vi "First Check.vi"(8 "error in (no error)":errorcluster) -> (0 "error out":errorcluster)   [LabVIEW 2023, in "Heart.lvlib"]
uses:
  Heart.lvlib
  <vilib>/xnet/xnet.llb/XNET Frame CAN.ctl
  <vilib>/xnet/xnet.llb/XNET Frame Type CAN.ctl
  <vilib>/xnet/xnet.llb/XNET Create Session (Frame Output Single-point).vi
  <vilib>/xnet/xnet.llb/XNET Create Session (Frame Input Single-point).vi
  <vilib>/xnet/xnet.llb/XNET Read (Frame CAN).vi
  <vilib>/xnet/xnet.llb/XNET Write (Frame CAN).vi
  Error Handling/Error Handling.lvlib
panel:
  out "Enter Manufactur Mode Frame Received":bool
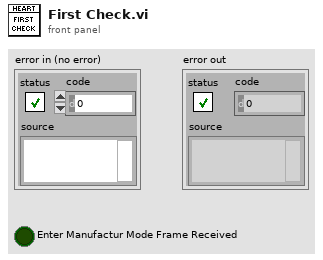
[diagram p1: front panel]
types:
  T1 = typedef "XNET Frame CAN.ctl" = cluster{"timestamp":timestamp, "payload":u8[], "identifier":u32, "type":T2, "extended?":bool, "echo?":bool}
  T2 = typedef "XNET Frame Type CAN.ctl" = u8
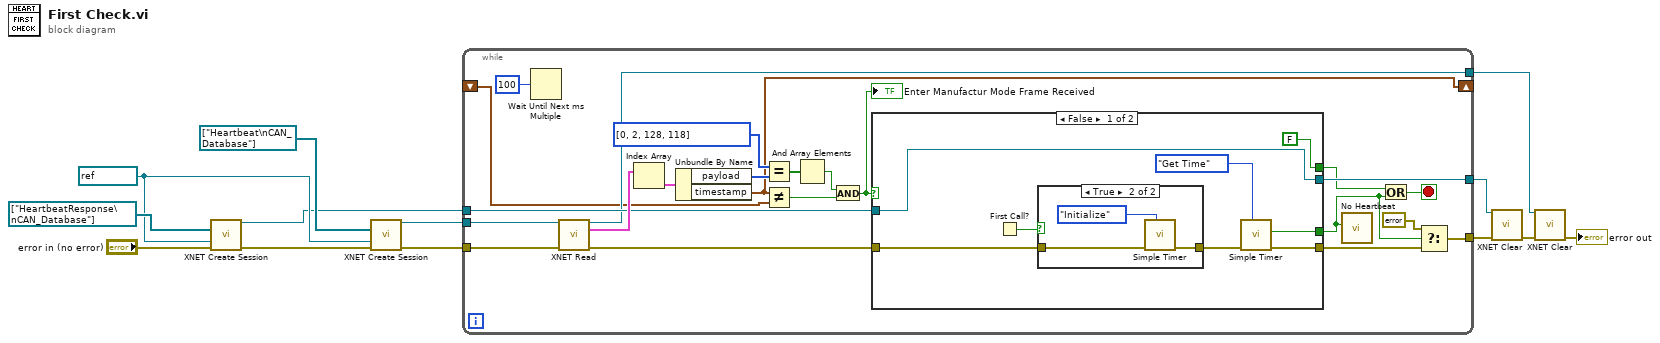
[diagram p0: block diagram]
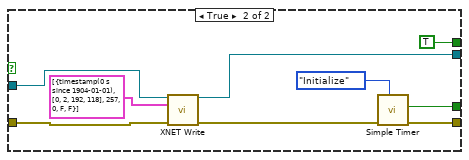
[diagram p3: hidden frame]
diagram:
  w8 = refnum<k21> "CAN2" ("interface")
  n1 = call-poly <vilib>:"XNET Create Session.vi"("frame list"=refnum<k21>[] ["HeartbeatResponse\nCAN_Database"], "interface"=w8, "error in (no error)"="error in (no error)") -> ("session out"=w7:refnum<k21>, "error out"=w6:errorcluster)  [unwired: 11 out]
  n2 = call-poly <vilib>:"XNET Create Session.vi"("frame list"=refnum<k21>[] ["Heartbeat\nCAN_Database"], "interface"=w8, "error in (no error)"=w6) -> ("session out"=w12:refnum<k21>, "error out"=w11:errorcluster)  [unwired: 11 out]
  n3 = while {
    tunnel: w12 -> [w36]
    tunnel: w11 -> [w35]
    tunnel: w7 -> [w31]
    tunnel: [w29] -> w1
    tunnel: [w20] -> w5
    tunnel: [w28] -> w2
    shift-right: [w17] -> _
    shift-left: _ -> [w16]
    stop <- w32 stop-if-true
    n4 = Wait Until Next ms Multiple(millisecond multiple=u32 100 ("milliseconds to wait")) -> ()  [unwired: 1 out]
    n5 = call-poly <vilib>:"XNET Read.vi"("session in"=w36, "error in (no error)"=w35) -> ("session out"=w29:refnum<k21>, "data"=w33:T1[], "error out"=w30:errorcluster)  [unwired: 11 out]
    n6 = Index Array(array=w33) -> (element=w23:T1)  [unwired: 1 in]
    n7 = Unbundle By Name(w23) -> ("payload"=w18:u8[], "timestamp"=w17:timestamp)
    n8 = Equal?(x=u8[] [0, 2, 128, 118] ("y"), y=w18) -> (x = y?=w25:bool[])
    n9 = Not Equal?(x=w17, y=w16) -> (x != y?=w27:bool)
    n10 = And Array Elements(Boolean array=w25) -> (logical AND=w24:bool)
    n11 = And(x=w24, y=w27) -> (x .and. y?=w26:bool)
    "Enter Manufactur Mode Frame Received" <- w26
    n12 = case shown="False" w26 {
      tunnel: [w43 w51] -> w15
      tunnel: w30 -> [w41 w55]
      tunnel: [w39 w56] -> w22
      tunnel: w31 -> [w38 w53]
      tunnel: [w38 w52] -> w28
      tunnel: [FALSE ("y") TRUE ("y")] -> w14
      frame False {
        n13 = First Call?() -> (First Call?: T/F=w42:bool)
        n14 = case shown="True" w42 {
          tunnel: w41 -> [w45 w47]
          tunnel: [w45 w46] -> w40
          frame False {
          }
          frame True {
            n15 = call "Simple Timer.vi"("Case Select"=enum16{"Get Time", "Initialize"}."Initialize", "Error in"=w47) -> ("error out"=w46:errorcluster)  [unwired: 7 in, 2 out]
          }
        }
        n16 = call "Simple Timer.vi"("Case Select"=enum16{"Get Time", "Initialize"}."Get Time", "Error in"=w40) -> ("error out"=w39:errorcluster, "Time Elapsed?"=w43:bool)  [unwired: 7 in, 1 out]
      }
      frame True {
        n17 = call-poly <vilib>:"XNET Write.vi"("session in"=w53, "data"=T1[] [{"timestamp"=timestamp(0 s since 1904-01-01), "payload"=[0, 2, 192, 118], "identifier"=257, "type"=0, "extended?"=FALSE, "echo?"=FALSE}], "error in (no error)"=w55) -> ("session out"=w52:refnum<k21>, "error out"=w54:errorcluster)  [unwired: 11 in]
        n18 = call "Simple Timer.vi"("Case Select"=enum16{"Get Time", "Initialize"}."Initialize", "Error in"=w54) -> ("error out"=w56:errorcluster, "Time Elapsed?"=w51:bool)  [unwired: 7 in, 1 out]
      }
    }
    n19 = call "No Heartbeat.vi"("No Heartbeat?"=w15) -> ()  [unwired: 10 in, 1 out]
    n20 = Or(x=w14, y=w15) -> (x .or. y?=w32:bool)
    n21 = Select(t=errorcluster {"status"=TRUE, "code"=69, "source"="No Heartbeat found on initial sequence"}, s=w15, f=w22) -> (s? t:f=w20:errorcluster)
  }
  n22 = call <vilib>:"XNET Clear.vi"("session in"=w2, "error in (no error)"=w5) -> ("error out"=w4:errorcluster)  [unwired: 13 in]
  n23 = call <vilib>:"XNET Clear.vi"("session in"=w1, "error in (no error)"=w4) -> ("error out"=→"error out":errorcluster)  [unwired: 13 in]
